vi "Configure Head Type.vi"(5 "Retry Attempts (0)":i32 min=0, 8 "error in":errorcluster, 10 "Head Type":i32, 11 "VISA resource name":refnum<visa-resource-name>) -> (0 "error out":errorcluster, 3 "VISA resource name out":refnum<visa-resource-name>)   [LabVIEW 2020, in "ChromTech Series III Pump.lvlib"]
doc: "Sets the pump head type, where:\n x = 1 for a stainless steel 10 mL/min pump head\n x = 2 for a plastic 10 mL/min pump head\n x = 3 for a stainless steel 40 mL/min pump head\n x = 4 for a plastic 40 mL/min pump head\nThe pump is stopped; and, the pressure compensation\nand pressure limits are initialized, when the head type is\nchanged.\nNote: This VI does not do error checking! Please consult the user manual to ensure the correct values are used."
uses:
  <instrlib>/RxnRover/ChromtechSeriesIIIDriver/ChromTech Series III Pump.lvlib
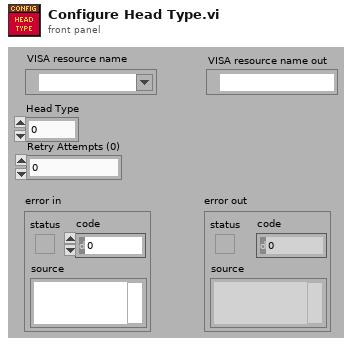
[diagram p1: front panel]
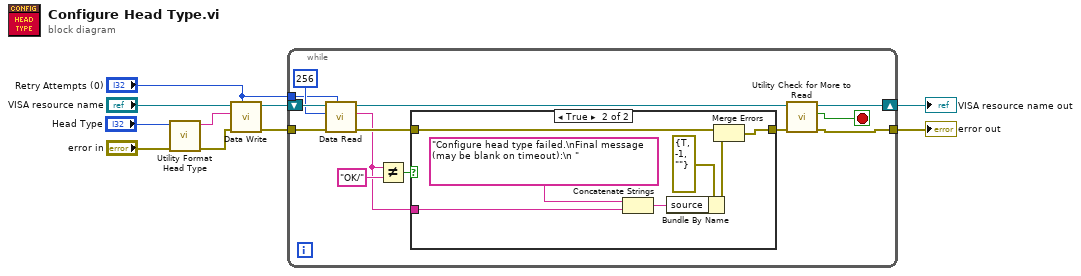
[diagram p0: block diagram]
diagram:
  n1 = call <instrlib>:"Utility Format Head Type.vi"("error in (no error)"="error in", "Head Type"="Head Type") -> ("error out"=w6:errorcluster, "Formatted Head Type"=w5:string)  [unwired: 8 in]
  n2 = call <instrlib>:"Data Write.vi"("Retry Attempts (0)"="Retry Attempts (0)", "error in (no error)"=w6, "Command"=w5, "VISA Refnum in"="VISA resource name") -> ("error out"=w9:errorcluster, "VISA Refnum out"=w4:refnum<visa-resource-name>)  [unwired: 6 in]
  n3 = while {
    tunnel: "Retry Attempts (0)" -> [w20]
    shift-right: [w12] -> w1
    shift-left: w4 -> [w22]
    tunnel: w9 -> [w23]
    tunnel: [w14] -> w2
    stop <- w11 stop-if-true
    n4 = call <instrlib>:"Data Read.vi"("Retry Attempts (0)"=w20, "error in (no error)"=w23, "Bytes to read"=256, "VISA Refnum in"=w22) -> ("error out"=w17:errorcluster, "read buffer"=w15:string, "VISA Refnum out"=w13:refnum<visa-resource-name>)  [unwired: 5 in]
    n5 = Not Equal?(x=w15, y="OK/") -> (x != y?=w18:bool)
    n6 = case shown="True" w18 {
      tunnel: [w24 w30] -> w16
      tunnel: w17 -> [w24 w29]
      tunnel: w15 -> [_ w25]
      frame False {
      }
      frame True {
        n7 = Concatenate Strings("Configure head type failed.\nFinal message (may be blank on timeout):\n ", w25) -> (w27:string)
        n8 = Bundle By Name(cluster=errorcluster {"status"=TRUE, "code"=-1, "source"=""} ("error out"), "source"=w27) -> (w28:errorcluster)
        n9 = Merge Errors(w29, w28) -> (w30:errorcluster)
      }
    }
    n10 = call <instrlib>:"Utility Check for More to Read.vi"("error in (no error)"=w16, "VISA Refnum in"=w13) -> ("error out (unchanged)"=w14:errorcluster, "More to read?"=w11:bool, "VISA Refnum out"=w12:refnum<visa-resource-name>)  [unwired: 7 in]
  }
  "VISA resource name out" <- w1
  "error out" <- w2
